vi "LinkUserEvent.vi"(8 "error in (no error)":errorcluster, 11 "Messenger in":refnum<class "MGR.lvclass">) -> (0 "error out":errorcluster, 2 "Messenger Event":refnum<user-event>, 3 "EventMessenger out":refnum<class "EventMessenger.lvclass">)   [LabVIEW 2011, in "Messenging.lvlib" / "LinkedEventMessenger.lvclass"]
uses:
  LinkedEventMessenger.lvclass
  Messenger (Parent)/MGR.lvclass
  TextVarientMessage/MSG.lvclass
  EventMessenger/EventMessenger.lvclass
  LinkedEventMessenger.lvclass/LinkedEventMessenger.ctl
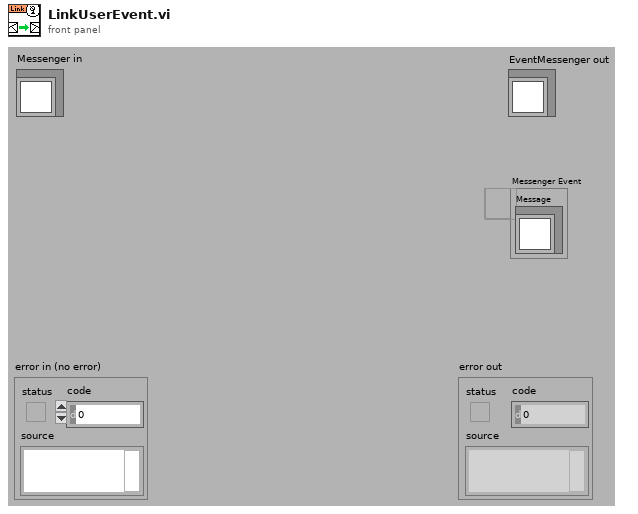
[diagram p1: front panel]
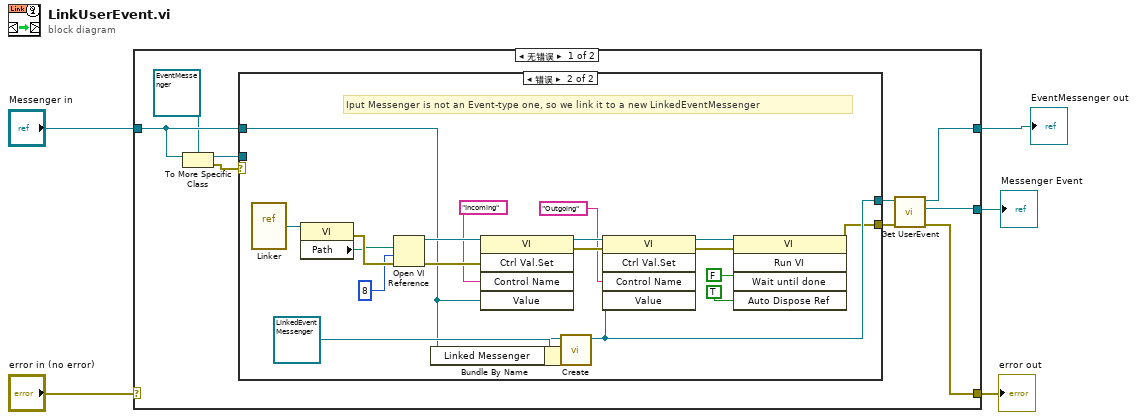
[diagram p0: block diagram]
diagram:
  n1 = case shown="无错误" "error in (no error)" {
    selector: "error in (no error)" -> [_ w35]
    tunnel: [w10 w35] -> w4
    tunnel: [w12 _] -> w1
    tunnel: "Messenger in" -> [w9 _]
    tunnel: [w13 _] -> w2
    frame No Error {
      n2 = To More Specific Class(target class=refnum<class "EventMessenger.lvclass"> refnum ("Event Messenger"), reference=w9) -> (specific class reference=w6:refnum<class "EventMessenger.lvclass">, error out=w7:errorcluster)  [unwired: 1 in]
      n3 = case shown="错误" w7 {
        tunnel: [w15 w20] -> w14
        tunnel: [_ w19] -> w11
        tunnel: w9 -> [_ w17]
        tunnel: w6 -> [w15 _]
        frame No Error {
          # "Input Messenger is already an Event-type messenger, so just use it as is"
        }
        frame Error {
          # "Iput Messenger is not an Event-type one, so we link it to a new LinkedEventMessenger"
          n4 = vi-ref "Linker.vi"() -> (w31:refnum<vi>)
          n5 = property class="VI"(reference=w31) -> (error out=w34:errorcluster, "Path"=w33:path)  [unwired: 1 in, 1 out]
          n6 = Open VI Reference(vi path=w33, options=8, error in (no error)=w34) -> (vi reference=w28:refnum<vi>, error out=w27:errorcluster)  [unwired: 1 in, 2 out]
          n7 = Bundle By Name(cluster=refnum<class "LinkedEventMessenger.lvclass"> refnum ("LinkedEventMessenger.lvclass"), "Linked Messenger"=w17) -> (w16:refnum<class "LinkedEventMessenger.lvclass">)
          n8 = invoke class="VI" method="Ctrl Val.Set"(reference=w28, error in=w27, "Control Name"="Incoming", "Value"=w17) -> (reference out=w25:refnum<vi>, error out=w24:errorcluster)  [unwired: 1 in, 3 out]
          n9 = call-dynamic "Create.vi"("EventMessenger in"=w16) -> ("EventMessenger out"=w20:refnum<class "LinkedEventMessenger.lvclass">)  [unwired: 1 in, 9 out]
          n10 = invoke class="VI" method="Ctrl Val.Set"(reference=w25, error in=w24, "Control Name"="Outgoing", "Value"=w20) -> (reference out=w22:refnum<vi>, error out=w21:errorcluster)  [unwired: 1 in, 3 out]
          n11 = invoke class="VI" method="Run VI"(reference=w22, error in=w21, "Wait until done"=FALSE ("Wait Until Done"), "Auto Dispose Ref"=TRUE ("Auto Dispose Reference")) -> (error out=w19:errorcluster)  [unwired: 1 in, 4 out]
        }
      }
      n12 = call-dynamic "Get UserEvent.vi"("error in"=w11, "EventMessenger"=w14) -> ("error out"=w10:errorcluster, "Messenger Event"=w13:refnum<user-event>, "EventMessenger out"=w12:refnum<class "EventMessenger.lvclass">)  [unwired: 7 out]
    }
    frame Error {
    }
  }
  "error out" <- w4
  "Messenger Event" <- w2
  "EventMessenger out" <- w1
